vi "Inst.Xeryon-Rotator.Set State.vi"(8 "error in (no error)":errorcluster, 10 "Scan State":T1, 11 "Inst.Xeryon-Rotator in":refnum<class "Inst.Xeryon-Rotator.lvclass">) -> (0 "error out":errorcluster, 3 "Inst.Xeryon-Rotator out":refnum<class "Inst.Xeryon-Rotator.lvclass">)   [LabVIEW 2019, in "Inst.Xeryon-Rotator.lvclass"]
uses:
  Inst.Xeryon-Rotator.lvclass
  Typedefs/Inst.Xeryon-Rotator.ScanState--Enum.ctl
  Inst.Xeryon-Rotator.lvclass/Inst.Xeryon-Rotator.ctl
  Controller.LV/Controller.LV.lvclass
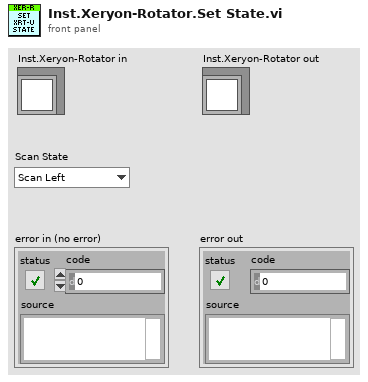
[diagram p1: front panel]
types:
  T1 = typedef "Inst.Xeryon-Rotator.lvclass/Inst.Xeryon-Rotator.ScanState--Enum.ctl" = enum16{"Scan Left", "Stop", "Scan Right", "Reset"}
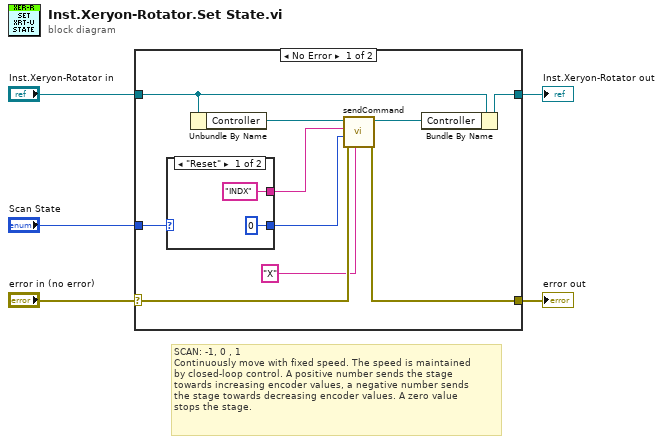
[diagram p0: block diagram]
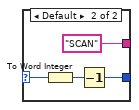
[diagram p2: hidden frame]
diagram:
  # "SCAN: -1, 0 , 1\nContinuously move with fixed speed. The speed is maintained\nby closed-loop control. A positive number sends the stage\ntowards increasing encoder values, a negative number sends\nthe stage towards decreasing encoder values. A zero value\nstops the stage."
  n1 = case shown="No Error" "error in (no error)" {
    selector: "error in (no error)" -> [w12 w23]
    tunnel: "Inst.Xeryon-Rotator in" -> [w14 w22]
    tunnel: [w11 w23] -> w3
    tunnel: "Scan State" -> [w6 _]
    tunnel: [w10 w22] -> w1
    frame No Error {
      n2 = case shown="\"Reset\"" w6 {
        selector: w6 -> [_ w18]
        tunnel: [i16 0 w20] -> w8
        tunnel: ["INDX" "SCAN"] -> w7
        frame "Reset" {
        }
        frame Default {
          n3 = To Word Integer(number=w18) -> (16bit integer=w21:i16)
          n4 = Decrement(x=w21) -> (x-1=w20:i16)
        }
      }
      n5 = Unbundle By Name(w14) -> ("Controller"=w15:refnum<class "Controller.LV.lvclass">)
      n6 = call-dynamic "sendCommand.vi"("Axis Letter"="X", "error in (no error)"=w12, "Value"=w8, "Command"=w7, "Controller in"=w15) -> ("error out"=w11:errorcluster, "Controller out"=w13:refnum<class "Controller.LV.lvclass">)  [unwired: 5 in]
      n7 = Bundle By Name(cluster=w14, "Controller"=w13) -> (w10:refnum<class "Inst.Xeryon-Rotator.lvclass">)
    }
    frame Error {
    }
  }
  "Inst.Xeryon-Rotator out" <- w1
  "error out" <- w3
